vi "WFRepetitions.vi"(9 "N":i32=1, 10 "Int (s)":dbl min=0.0 format="%#_4g", 11 "Del (s)":dbl min=0.0 format="%#_4f") -> (3 "WFRepetitions":T1={"Del (s)"=100000.0, "Int (s)"=1.0, "N"=0} {"Int (s)" min=0.0 format="%#_4g"; "Del (s)" min=0.0 format="%#_4f"})   [LabVIEW 2013]
uses:
  WFRepetitions.ctl
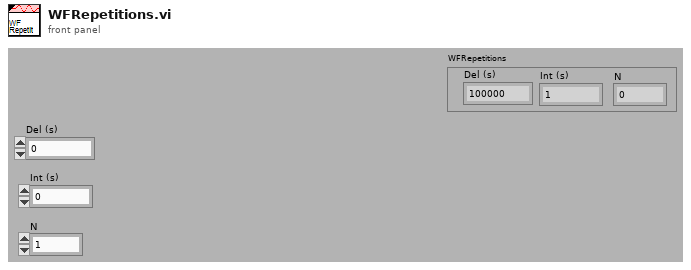
[diagram p1: front panel]
types:
  T1 = typedef "WFRepetitions.ctl" = cluster{"Del (s)":dbl, "Int (s)":dbl, "N":i32}
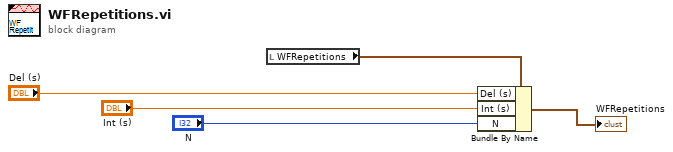
[diagram p0: block diagram]
diagram:
  n1 = local read "WFRepetitions"() -> (w4:T1)
  n2 = Bundle By Name(cluster=w4, "Del (s)"="Del (s)", "Int (s)"="Int (s)", "N"="N") -> (→"WFRepetitions":T1)
